vi "Trajectory_lerp_double.vi"(9 "fraction":dbl, 10 "endValue":dbl, 11 "startValue":dbl) -> (3 "outputValue":dbl)   [LabVIEW 2019, in "Trajectory_Library.lvlib"]
doc: "This is an internal routine. Linearly interpolates between two values.\n\nParameters:\n - startValue - The start value.\n - endValue - The end value.\n - fraction - The fraction for interpolation.\n\nReturn:\n - outputValue - The interpolated value."
uses:
  Trajectory_Library.lvlib
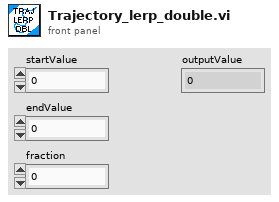
[diagram p1: front panel]
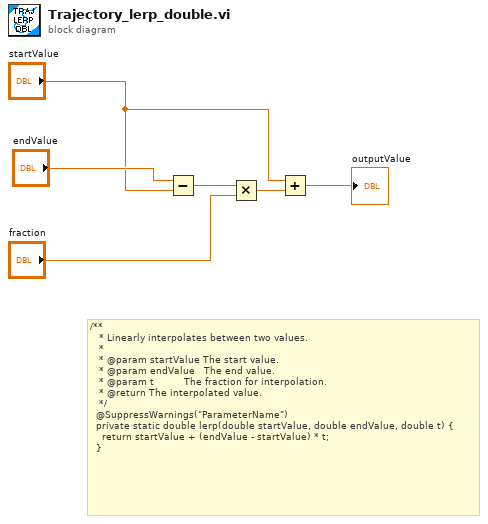
[diagram p0: block diagram]
diagram:
  # "/**\n   * Linearly interpolates between two values.\n   *\n   * @param startValue The start value.\n   * @param endValue   The end value.\n   * @param t          The fraction for interpolation.\n   * @return The interpolated value.\n   */\n  @SuppressWarnings(\"ParameterName\")\n  private static double lerp(double startValue, double endValue, double t) {\n    return startValue + (endValue - startValue) * t;\n  }"
  n1 = Subtract(x="endValue", y="startValue") -> (x-y=w5:dbl)
  n2 = Multiply(x=w5, y="fraction") -> (x*y=w3:dbl)
  n3 = Add(x="startValue", y=w3) -> (x+y=→"outputValue":dbl)
